vi "FTW-FileSystem-OpenURIwithDefaultHandler.vi"(0 "URI to Open":string, 11 "error in":errorcluster) -> (4 "URI Actually Opened":string, 15 "error out":errorcluster)   [LabVIEW 2012]
panel:
  # "Inputs"
  # "Outputs"
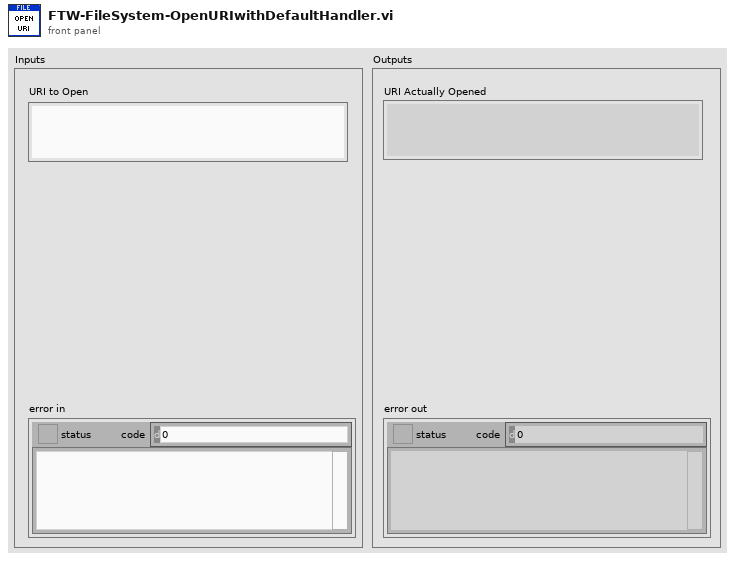
[diagram p1: front panel]
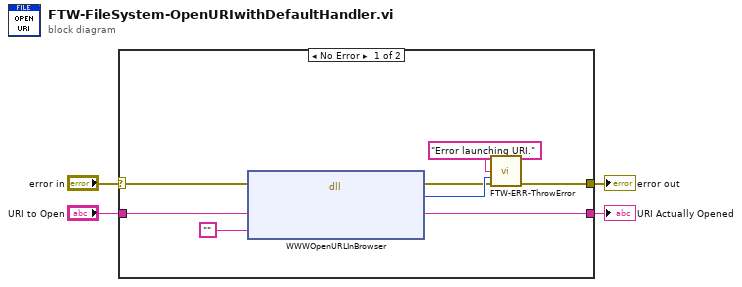
[diagram p0: block diagram]
diagram:
  n1 = case shown="No Error" "error in" {
    selector: "error in" -> [w9 w13]
    tunnel: "URI to Open" -> [w12 _]
    tunnel: [w11 _] -> w3
    tunnel: [w6 w13] -> w1
    frame No Error {
      n2 = dll-call lib="LabVIEW" fn="WWWOpenURLInBrowser"(error in=w9, "URI"=w12, "BrowserPath"="") -> (error out=w7:errorcluster, "Error Code"=w8:i32, "URI"=w11:string)  [unwired: 3 in, 1 out]
      n3 = call "FTW-ERR-ThrowError.vi"("Error Message"="Error launching URI.", "Error Code"=w8, "error in"=w7) -> ("error out"=w6:errorcluster)  [unwired: 12 in]
    }
    frame Error {
    }
  }
  "error out" <- w1
  "URI Actually Opened" <- w3
